vi "GlobalVar.vi"() -> ()   [LabVIEW 2012]
panel:
  in  "9220/AI0":fxp<+/-,24,5>
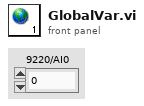
[diagram p1: front panel]
diagram:
